vi "check syntax_core.vi"(8 "error in (no error)":errorcluster caption="에러 입력(에러 없음)", 11 "Script Line_delay 입력":refnum<class "Script Line_delay.lvclass">) -> (0 "error out":errorcluster caption="에러 출력", 3 "Script Line_delay 출력":refnum<class "Script Line_delay.lvclass">)   [LabVIEW 2020, in "Script Line_delay.lvclass"]
uses:
  Script Line_delay.lvclass
  Script Line/Script Line.lvclass/Script Line.ctl
  Script Line_delay.lvclass/Script Line_delay.ctl
  Script Line/Accessors/Read parameter.vi
  Script Line/Accessors/Read parameter string index.vi
  Script Line/Script Line.lvclass
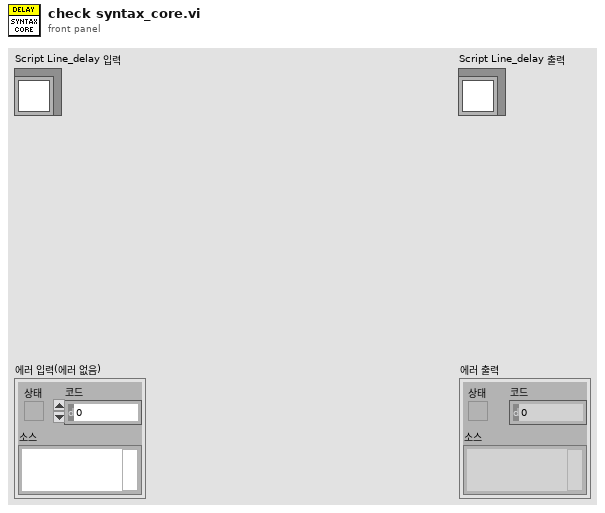
[diagram p1: front panel]
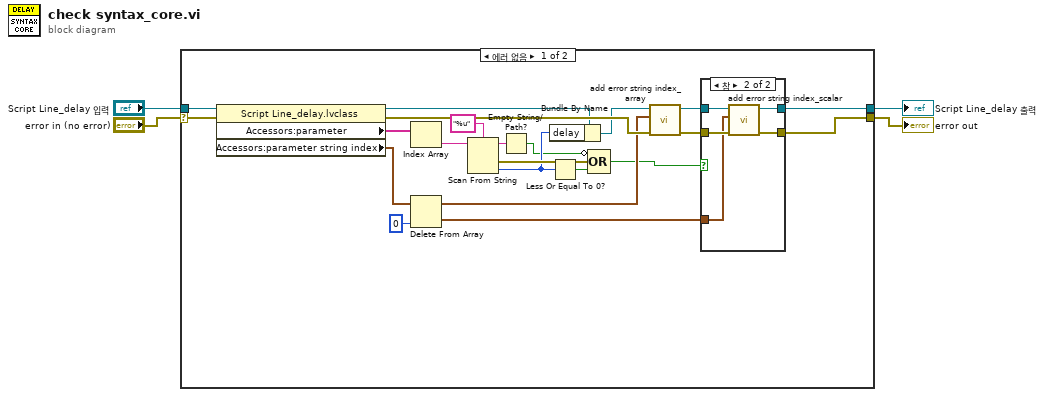
[diagram p0: block diagram]
diagram:
  n1 = case shown="에러 없음" "error in (no error)" {
    selector: "error in (no error)" -> [w25 w35]
    tunnel: [w15 w35] -> w4
    tunnel: [w13 w34] -> w3
    tunnel: "Script Line_delay 입력" -> [w26 w34]
    frame No Error {
      n2 = property class="Script Line_delay.lvclass"(reference=w26, error in=w25) -> (reference out=w9:refnum<class "Script Line_delay.lvclass">, error out=w24:errorcluster, "Accessors:parameter"=w23:string[], "Accessors:parameter string index"=w10:cluster{"start":u32, "end":u32}[])
      n3 = Index Array(array=w23) -> (element=w22:string)  [unwired: 1 in]
      n4 = Delete From Array(array=w10, index=0 ("인덱스")) -> (deleted portion=w12:cluster{"start":u32, "end":u32}, array with subset deleted=w16:cluster{"start":u32, "end":u32}[])  [unwired: 1 in]
      n5 = Scan From String(format string="%u" ("포맷 문자열"), input string=w22) -> (remaining string=w6:string, error out=w20:errorcluster, output 1=w8:u32)  [unwired: 3 in, 1 out]
      n6 = Empty String/Path?(string/path=w6) -> (empty?=w5:bool)
      n7 = Bundle By Name(cluster=w9, "delay"=w8) -> (w7:refnum<class "Script Line_delay.lvclass">)
      n8 = Less Or Equal To 0?(x=w8) -> (x <= 0?=w19:bool)
      n9 = Compound Arithmetic op=OR(invert w5, w20, w19) -> (w11:bool)
      n10 = call "add error string index_array.vi"("error in (no error)"=w24, "index_array"=w16, "Script Line 입력"=w7) -> ("error out"=w18:errorcluster, "Script Line 출력"=w14:refnum<class "Script Line_delay.lvclass">)  [unwired: 7 in]
      n11 = case shown="참" w11 {
        tunnel: w18 -> [w27 w33]
        tunnel: [w27 w32] -> w15
        tunnel: w14 -> [w28 w31]
        tunnel: [w28 w30] -> w13
        tunnel: w12 -> [_ w29]
        frame False {
        }
        frame True {
          n12 = call "add error string index_scalar.vi"("error in (no error)"=w33, "index_scalar"=w29, "Script Line 입력"=w31) -> ("error out"=w32:errorcluster, "Script Line 출력"=w30:refnum<class "Script Line_delay.lvclass">)  [unwired: 7 in]
        }
      }
    }
    frame Error {
    }
  }
  "error out" <- w4
  "Script Line_delay 출력" <- w3
